vi "Destroy REST Client.vi"(8 "error in (no error)":errorcluster, 11 "REST Client in":refnum<class "REST Client_JKI.lvclass">) -> (0 "error out":errorcluster)   [LabVIEW 2018, in "REST Client.lvlib" / "REST Client_JKI.lvclass"]
doc: "Destroy REST client reference."
uses:
  REST Client_JKI.lvclass
  REST Client_JKI.lvclass/REST Client_JKI.ctl
  <vilib>/httpClient/LabVIEWHTTPClient.lvlib
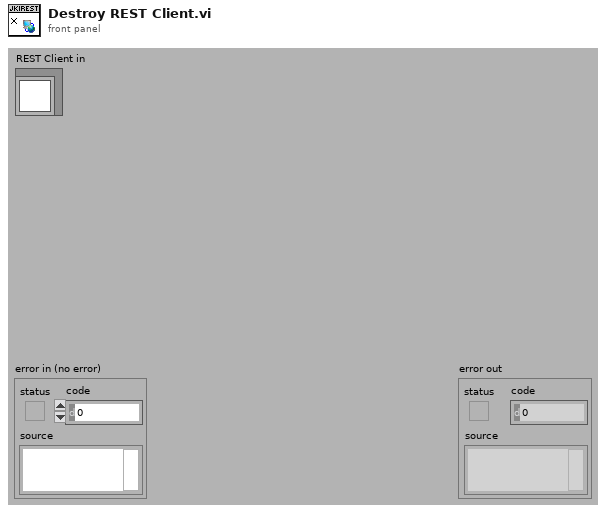
[diagram p1: front panel]
types:
  T1 = typedef "LabVIEWHTTPClient.lvlib/ClientHandle.ctl" = refnum<k1>
  T2 = typedef "REST Client.lvlib/REST Client.lvclass/HTTP Header.ctl" = cluster{"header":string, "value":string}
  T3 = cluster{"client handle out":T1, "Default Headers ([JSON])":T2[]}[]
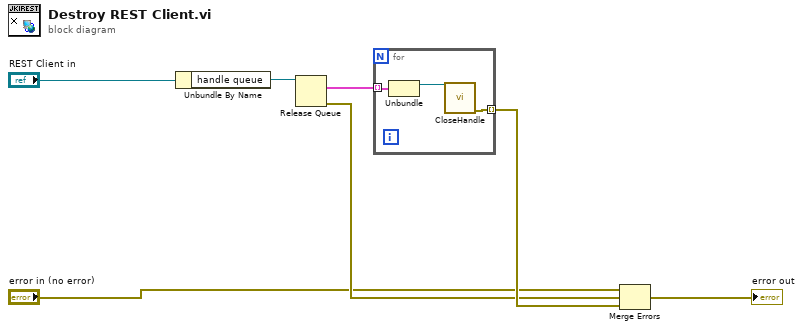
[diagram p0: block diagram]
diagram:
  n1 = Unbundle By Name("REST Client in") -> ("handle queue"=w6:refnum<queue>)
  n2 = Release Queue(queue=w6) -> (remaining elements=w5:T3, error out=w2:errorcluster)  [unwired: 2 in, 1 out]
  n3 = for {
    tunnel: w5 -> [w9] mode=indexing
    tunnel: [w10] -> w3 mode=indexing
    n4 = Unbundle(w9) -> ("client handle out"=w8:T1)  [unwired: 1 out]
    n5 = call <vilib>:"CloseHandle.vi"("client handle"=w8) -> ("error out"=w10:errorcluster)  [unwired: 14 in]
  }
  n6 = Merge Errors("error in (no error)", w2, w3) -> (→"error out":errorcluster)
